vi "FGV_Dot_NET_Root_Node.vi"(7 "Action":enum16{"Set", "Get"}(ring), 8 "error in (no error)":errorcluster, 11 "GetNodeRoot":refnum<k24>) -> (0 "error out":errorcluster, 3 "GetNodeRoot 2":refnum<k24>)   [LabVIEW 2013]
uses:
  NationalInstruments.VeriStand.SystemStorage
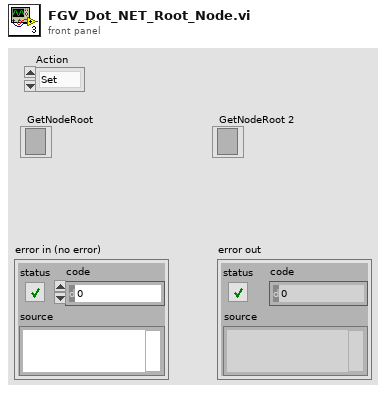
[diagram p1: front panel]
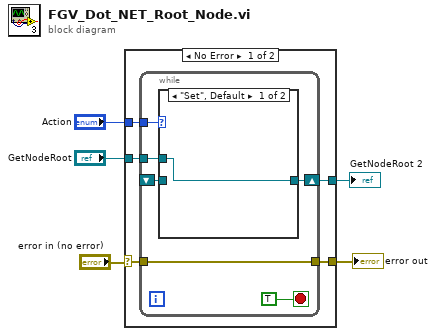
[diagram p0: block diagram]
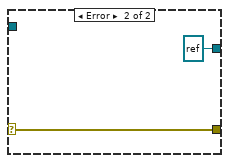
[diagram p3: hidden frame]
diagram:
  n1 = case shown="No Error" "error in (no error)" {
    selector: "error in (no error)" -> [w10 w20]
    tunnel: [w6 w20] -> w4
    tunnel: "Action" -> [w9 _]
    tunnel: "GetNodeRoot" -> [w8 _]
    tunnel: [w7 refnum<k24> refnum ("GetNodeRoot")] -> w1
    frame No Error {
      n2 = while {
        tunnel: w10 -> [w11]
        tunnel: w9 -> [w15]
        tunnel: w8 -> [w14]
        shift-right: [w13] -> w7
        shift-left: _ -> [w12]
        tunnel: [w11] -> w6
        stop <- TRUE stop-if-true
        n3 = case shown="\"Set\", Default" w15 {
          tunnel: w14 -> [w17 _]
          tunnel: [w17 w18] -> w13
          tunnel: w12 -> [_ w18]
          frame "Set", Default {
          }
          frame "Get" {
          }
        }
      }
    }
    frame Error {
    }
  }
  "error out" <- w4
  "GetNodeRoot 2" <- w1
